vi "2B_Tech_TCP_Packet_CABOZO_v1.1.vi"(7 "TCP Packet In":string, 12 "Data Array":string[](array[string])) -> (8 "TCP Binary Packet":string)   [LabVIEW 2014]
panel:
  out "array":string[](array[string])
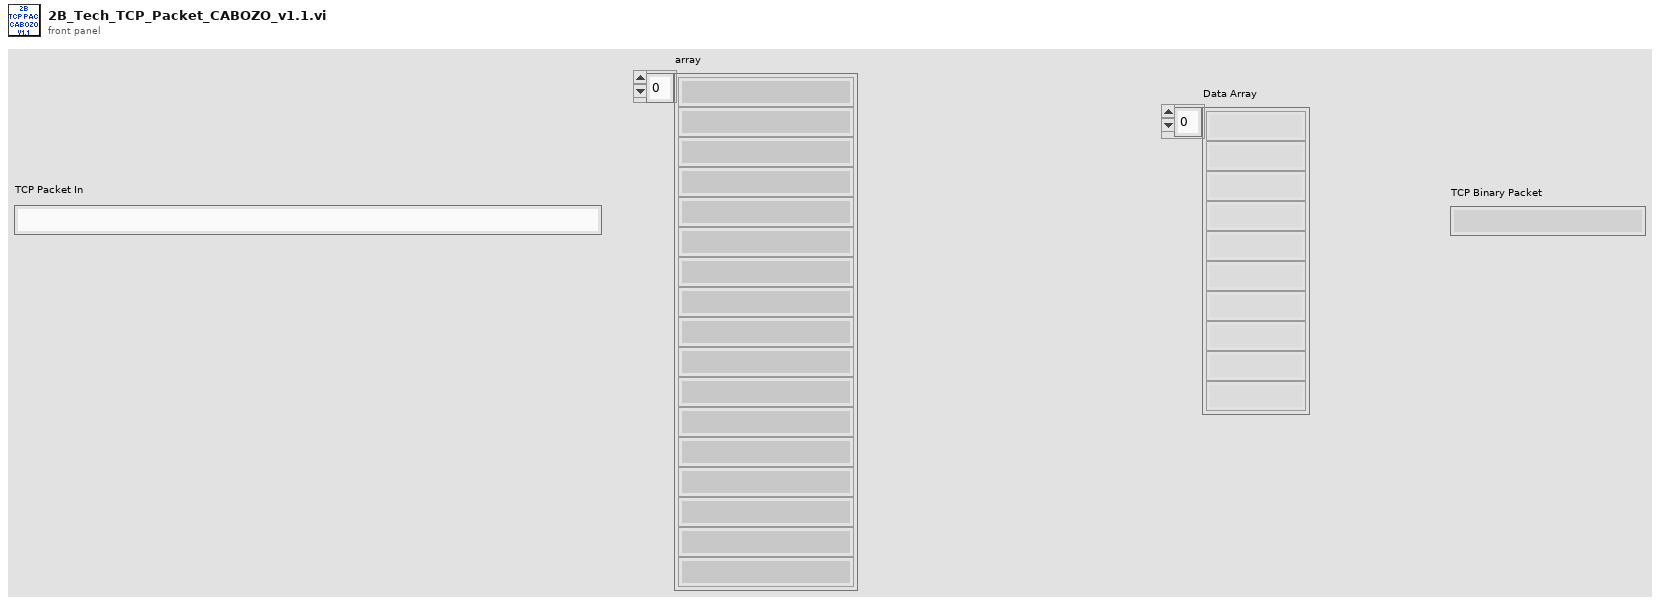
[diagram p1: front panel]
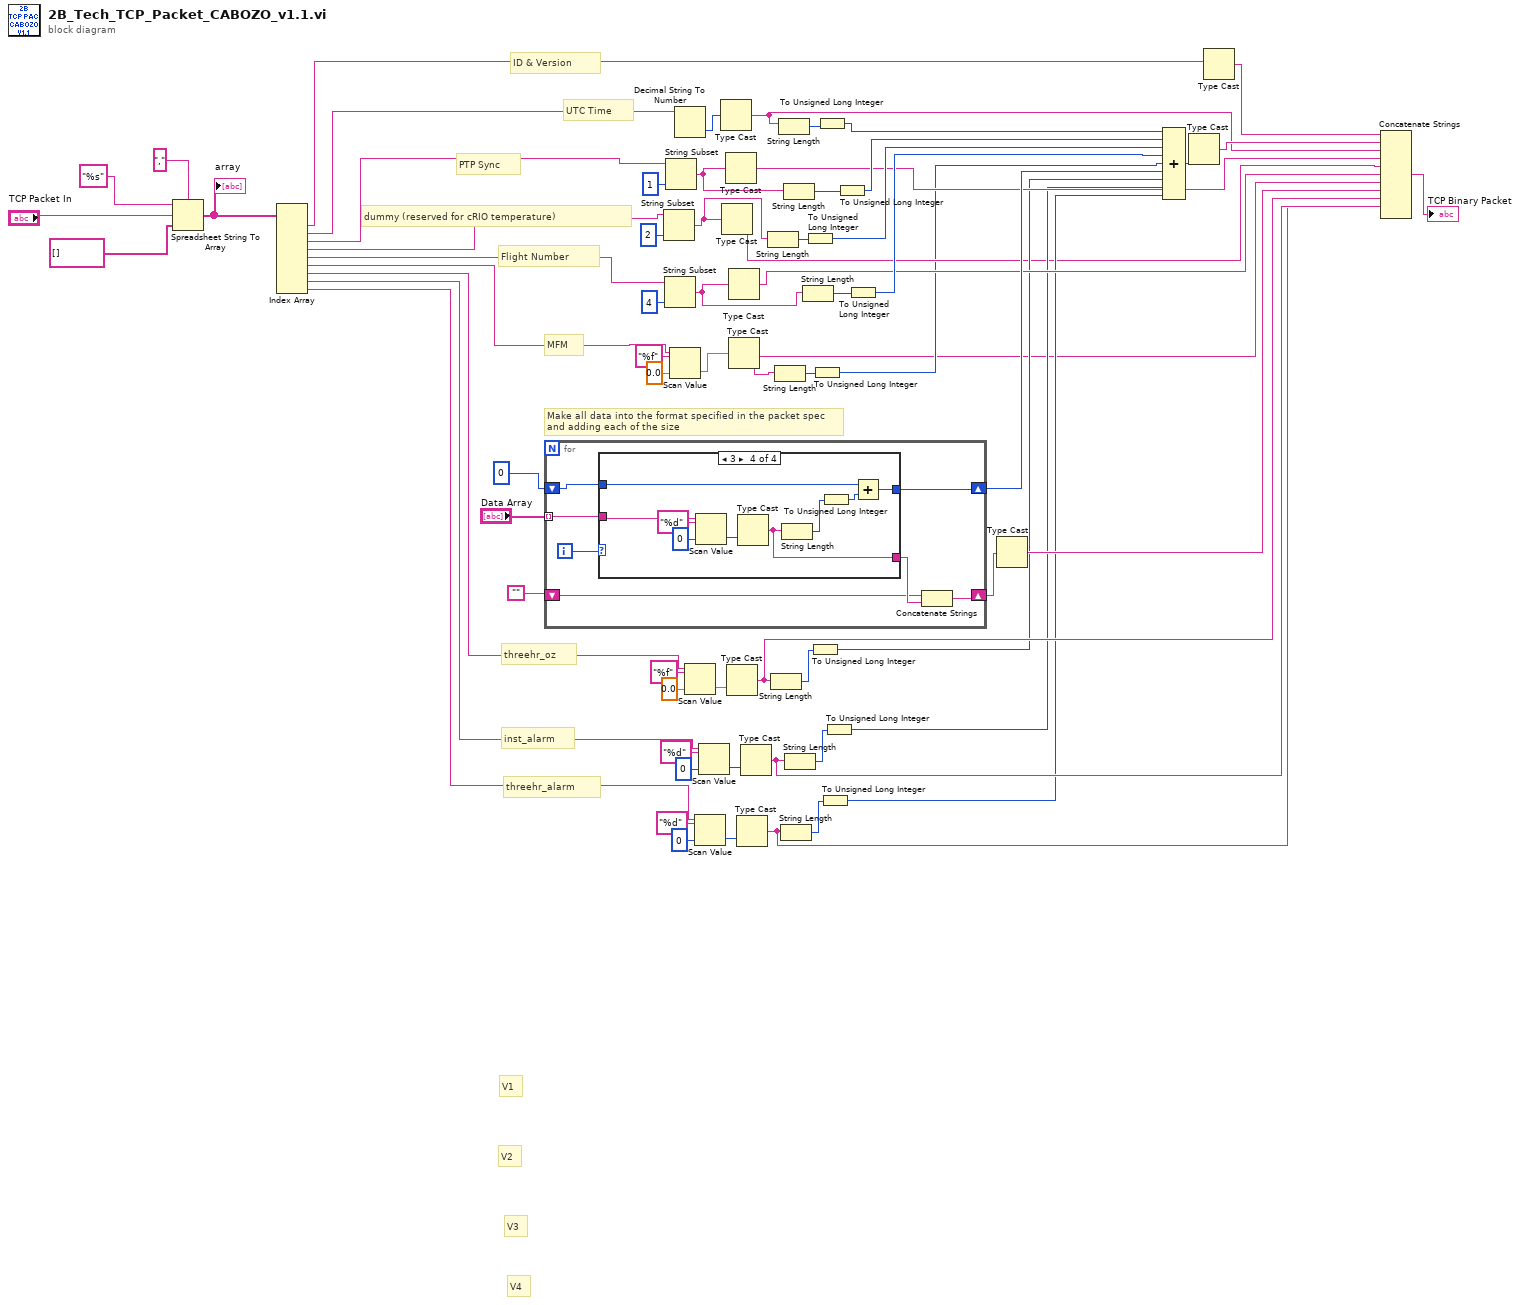
[diagram p0: block diagram]
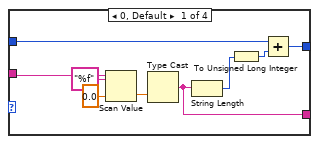
[diagram p2: hidden frame]
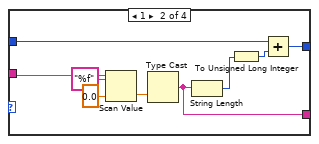
[diagram p3: hidden frame]
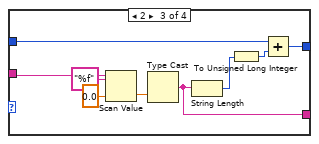
[diagram p4: hidden frame]
diagram:
  # "dummy (reserved for cRIO temperature)"
  # "V4"
  # "V3"
  # "V2"
  # "V1"
  # "threehr_alarm"
  # "inst_alarm"
  # "threehr_oz"
  # "Flight Number"
  # "MFM"
  # "PTP Sync"
  # "UTC Time"
  # "ID & Version"
  # "Make all data into the format specified in the packet spec\nand adding each of the size"
  n1 = Spreadsheet String To Array(delimiter (Tab)=",", format string="%s", spreadsheet string="TCP Packet In", array type (2D Dbl)=string[] []) -> (array=w27:string[])
  "array" <- w27
  n2 = Index Array(array=w27) -> (element #1=w26:string, element #2=w2:string, element #3=w25:string, element #4=w5:string, element #5=w24:string, element #6=w9:string, element #7=w14:string, element #8=w15:string, element #9=w16:string)  [unwired: 9 in]
  n3 = for {
    tunnel: "Data Array" -> [w73] mode=indexing
    shift-right: [w71] -> w55
    shift-left: u32 0 -> [w72]
    shift-right: [w70] -> w44
    shift-left: "" -> [w68]
    i -> [w74]
    n4 = case shown="3" w74 {
      tunnel: w73 -> [w81 w90 w99 w108]
      tunnel: w72 -> [w79 w88 w97 w106]
      tunnel: [w76 w85 w94 w103] -> w71
      tunnel: [w75 w84 w93 w102] -> w69
      frame 0, Default {
        n5 = Scan Value(string=w81, format string="%f", default (0 dbl)=sgl 0.0 ("default (0 I32)")) -> (value=w83:sgl)  [unwired: 1 out]
        n6 = Type Cast(x=w83) -> (*(type *) &x=w75:string)  [unwired: 1 in]
        n7 = String Length(string=w75) -> (length=w78:i32)
        n8 = To Unsigned Long Integer(number=w78) -> (unsigned 32bit integer=w77:u32)
        n9 = Add(x=w79, y=w77) -> (x+y=w76:u32)
      }
      frame 1 {
        n10 = Scan Value(string=w90, format string="%f", default (0 dbl)=sgl 0.0 ("default (0 I32)")) -> (value=w92:sgl)  [unwired: 1 out]
        n11 = Type Cast(x=w92) -> (*(type *) &x=w84:string)  [unwired: 1 in]
        n12 = String Length(string=w84) -> (length=w87:i32)
        n13 = To Unsigned Long Integer(number=w87) -> (unsigned 32bit integer=w86:u32)
        n14 = Add(x=w88, y=w86) -> (x+y=w85:u32)
      }
      frame 2 {
        n15 = Scan Value(string=w99, format string="%f", default (0 dbl)=sgl 0.0 ("default (0 I32)")) -> (value=w101:sgl)  [unwired: 1 out]
        n16 = Type Cast(x=w101) -> (*(type *) &x=w93:string)  [unwired: 1 in]
        n17 = String Length(string=w93) -> (length=w96:i32)
        n18 = To Unsigned Long Integer(number=w96) -> (unsigned 32bit integer=w95:u32)
        n19 = Add(x=w97, y=w95) -> (x+y=w94:u32)
      }
      frame 3 {
        n20 = Scan Value(string=w108, format string="%d", default (0 dbl)=0 ("default (0 I32)")) -> (value=w110:i32)  [unwired: 1 out]
        n21 = Type Cast(x=w110) -> (*(type *) &x=w102:string)  [unwired: 1 in]
        n22 = String Length(string=w102) -> (length=w105:i32)
        n23 = To Unsigned Long Integer(number=w105) -> (unsigned 32bit integer=w104:u32)
        n24 = Add(x=w106, y=w104) -> (x+y=w103:u32)
      }
    }
    n25 = Concatenate Strings(w68, w69) -> (w70:string)
  }
  n26 = String Subset(string=w5, length (rest)=2 ("length (rest)")) -> (substring=w4:string)  [unwired: 1 in]
  n27 = String Subset(string=w24, length (rest)=4 ("length (rest)")) -> (substring=w48:string)  [unwired: 1 in]
  n28 = String Subset(string=w25, length (rest)=1 ("length (rest)")) -> (substring=w51:string)  [unwired: 1 in]
  n29 = Scan Value(string=w9, format string="%f", default (0 dbl)=sgl 0.0 ("default (0 I32)")) -> (value=w10:sgl)  [unwired: 1 out]
  n30 = Decimal String To Number(string=w2) -> (number=w3:i32)  [unwired: 2 in, 1 out]
  n31 = Scan Value(string=w14, format string="%f", default (0 dbl)=sgl 0.0 ("default (0 I32)")) -> (value=w43:sgl)  [unwired: 1 out]
  n32 = Scan Value(string=w16, format string="%d", default (0 dbl)=u16 0 ("default (0 I32)")) -> (value=w23:u16)  [unwired: 1 out]
  n33 = Scan Value(string=w15, format string="%d", default (0 dbl)=u16 0 ("default (0 I32)")) -> (value=w37:u16)  [unwired: 1 out]
  n34 = Type Cast(x=w3) -> (*(type *) &x=w1:string)  [unwired: 1 in]
  n35 = Type Cast(x=w4) -> (*(type *) &x=w17:string)  [unwired: 1 in]
  n36 = Type Cast(x=w51) -> (*(type *) &x=w50:string)  [unwired: 1 in]
  n37 = Type Cast(x=w43) -> (*(type *) &x=w39:string)  [unwired: 1 in]
  n38 = Type Cast(x=w48) -> (*(type *) &x=w49:string)  [unwired: 1 in]
  n39 = Type Cast(x=w10) -> (*(type *) &x=w7:string)  [unwired: 1 in]
  n40 = Type Cast(x=w23) -> (*(type *) &x=w18:string)  [unwired: 1 in]
  n41 = Type Cast(x=w37) -> (*(type *) &x=w32:string)  [unwired: 1 in]
  n42 = String Length(string=w4) -> (length=w62:i32)
  n43 = String Length(string=w39) -> (length=w40:i32)
  n44 = String Length(string=w7) -> (length=w13:i32)
  n45 = String Length(string=w1) -> (length=w67:i32)
  n46 = String Length(string=w18) -> (length=w20:i32)
  n47 = String Length(string=w51) -> (length=w64:i32)
  n48 = String Length(string=w32) -> (length=w34:i32)
  n49 = String Length(string=w48) -> (length=w59:i32)
  n50 = To Unsigned Long Integer(number=w62) -> (unsigned 32bit integer=w61:u32)
  n51 = To Unsigned Long Integer(number=w40) -> (unsigned 32bit integer=w38:u32)
  n52 = To Unsigned Long Integer(number=w13) -> (unsigned 32bit integer=w8:u32)
  n53 = To Unsigned Long Integer(number=w67) -> (unsigned 32bit integer=w66:u32)
  n54 = To Unsigned Long Integer(number=w20) -> (unsigned 32bit integer=w19:u32)
  n55 = To Unsigned Long Integer(number=w34) -> (unsigned 32bit integer=w33:u32)
  n56 = To Unsigned Long Integer(number=w64) -> (unsigned 32bit integer=w63:u32)
  n57 = To Unsigned Long Integer(number=w59) -> (unsigned 32bit integer=w58:u32)
  n58 = Type Cast(x=w44) -> (*(type *) &x=w47:string)  [unwired: 1 in]
  n59 = Compound Arithmetic op=ADD(w66, w63, w61, w58, w8, w55, w38, w33, w19) -> (w53:u32)
  n60 = Type Cast(x=w53) -> (*(type *) &x=w52:string)  [unwired: 1 in]
  n61 = Type Cast(x=w26) -> (*(type *) &x=w54:string)  [unwired: 1 in]
  n62 = Concatenate Strings(w54, w52, w1, w50, w17, w49, w7, w47, w39, w32, w18) -> (→"TCP Binary Packet":string)
